vi "AMI_CREA_SECUENCIA_REPITE_NSCAN.vi"(8 "error in (no error)":errorcluster) -> (0 "error out":errorcluster, 3 "SECUENCIA":string[](array[string]), 4 "TOTAL_REPS":string[](array[string]), 6 "PASOS_REPS":i32)   [LabVIEW 2017]
uses:
  <vilib>/Utility/file.llb/Read Delimited Spreadsheet (string).vi
panel:
  out "Array 2":string[](array[string])
  out "PASOS":i32
  out "TOTAL":string[](array[string])
  out "Array":string[][][](array[string])
  out "PASOS_SECUENCIA":i32
  out "End_idx":i32[](array[numeric])
  out "Start_idx":i32[](array[numeric])
  out "Scan X":bool
  out "Scan Y":bool
  out "Scan V":bool
  out "Array2D":string[][](array[string])
  out "Scan T":bool
  out "Scan Z":bool
  in  "Salir":bool
  in  "Borrar línea":bool
  in  "Grabar":bool
  in  "Cargar":bool
  out "SequenceFile":path
  in  "Añadir: (doble click)":i32(listbox) caption="Válvulas"
  in  "Secuencia":i32(listbox)=-1
  # "Ene 2023 V1.6  a_sslcdms"
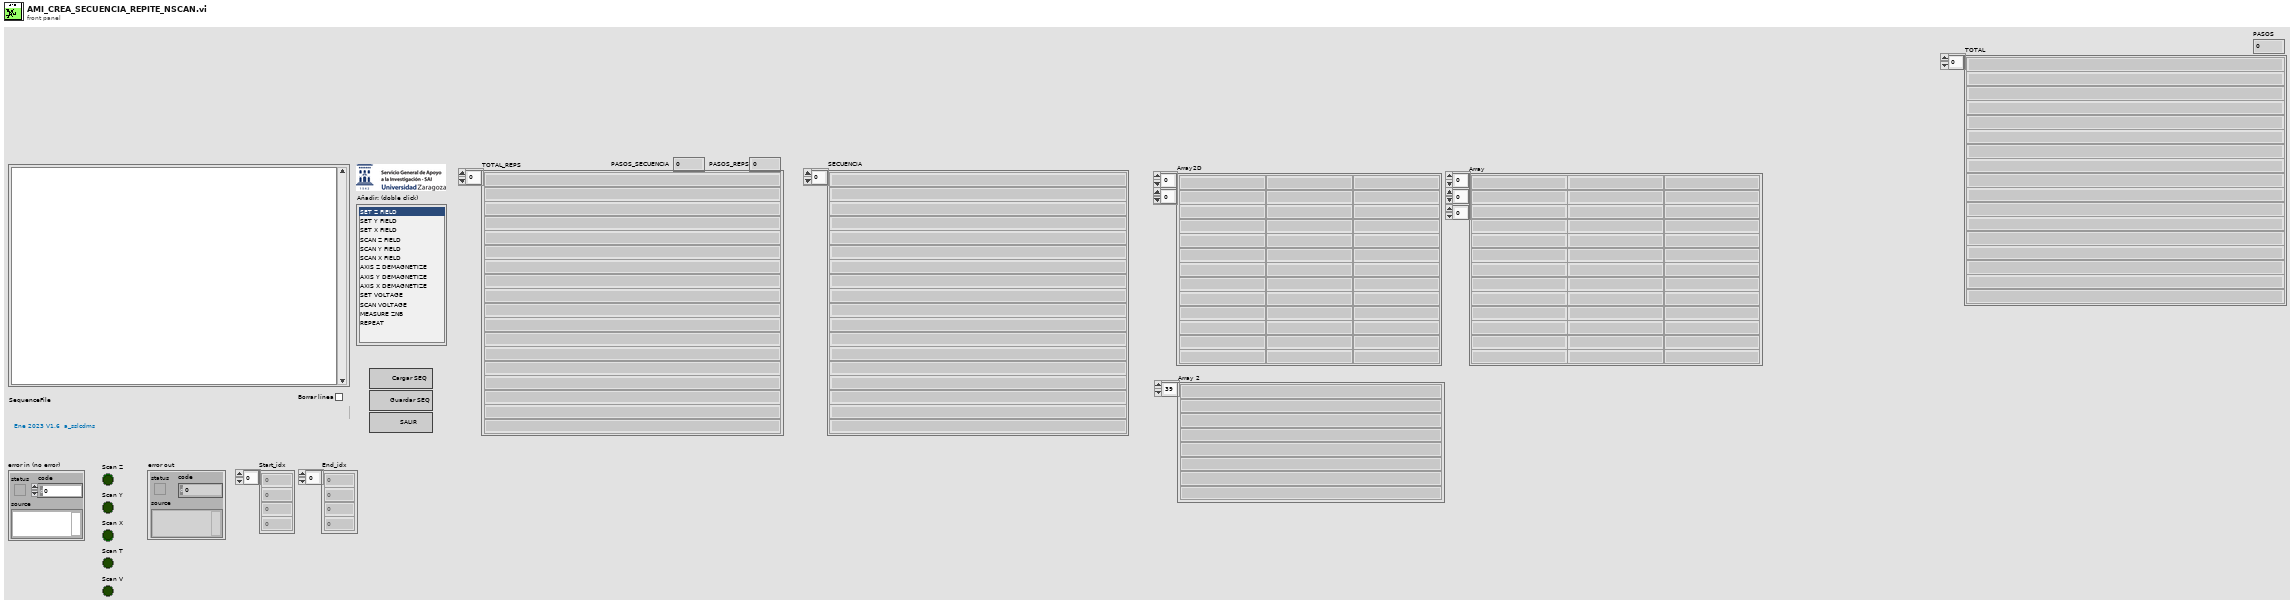
[diagram p1: front panel]
types:
  T1 = enum16{"open", "open or create", "create or replace", "create", "open (read only)"}
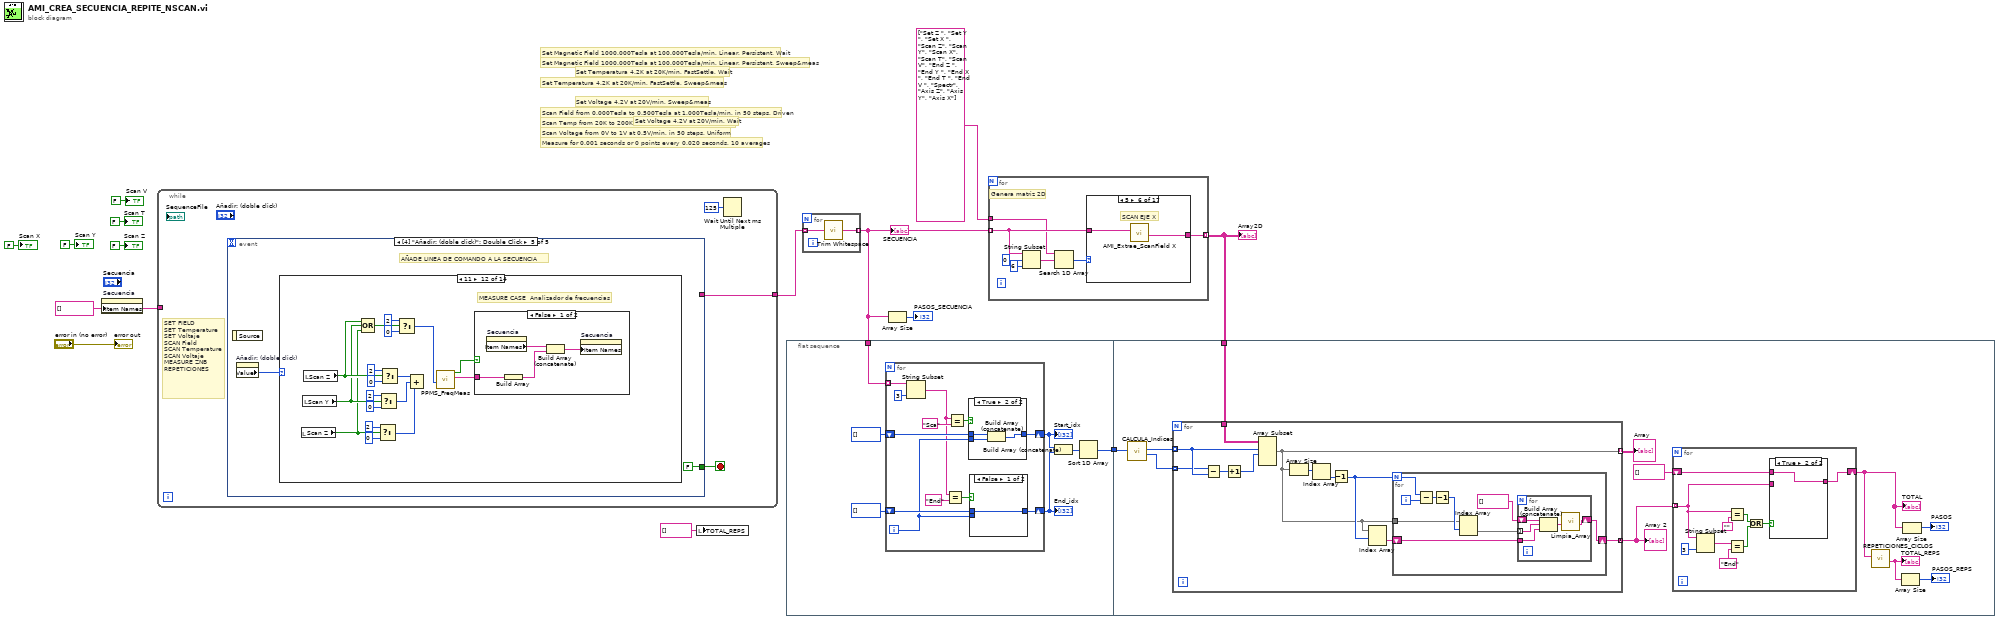
[diagram p0: block diagram]
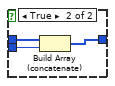
[diagram p2: hidden frame]
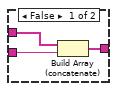
[diagram p4: hidden frame]
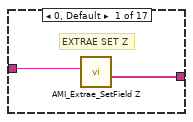
[diagram p5: hidden frame]
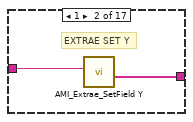
[diagram p6: hidden frame]
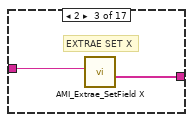
[diagram p7: hidden frame]
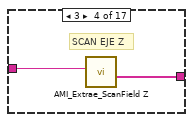
[diagram p8: hidden frame]
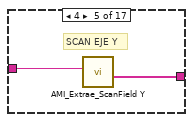
[diagram p9: hidden frame]
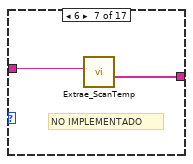
[diagram p10: hidden frame]
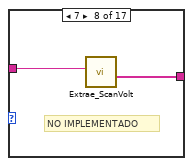
[diagram p11: hidden frame]
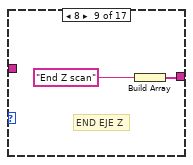
[diagram p12: hidden frame]
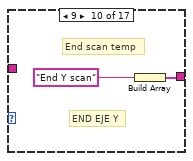
[diagram p13: hidden frame]
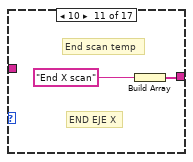
[diagram p14: hidden frame]
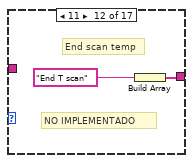
[diagram p15: hidden frame]
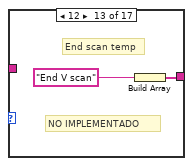
[diagram p16: hidden frame]
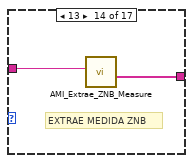
[diagram p17: hidden frame]
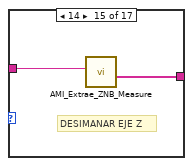
[diagram p18: hidden frame]
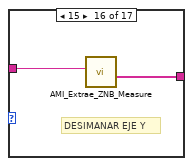
[diagram p19: hidden frame]
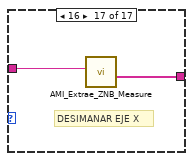
[diagram p20: hidden frame]
diagram:
  w14 = string[] [] ("Item Names")
  # "Measure for 0.001 seconds or 0 points every 0.020 seconds, 10 averages"
  # "Scan Voltage from 0V to 1V at 0.5V/min, in 50 steps, Uniform"
  # "Scan Temp from 20K to 200K at 0.1K/min, in 50 steps, Uniform"
  # "Scan Field from 0.000Tesla to 0.500Tesla at 1.000Tesla/min, in 50 steps, Driven"
  # "Set Temperatura 4.2K at 20K/min, FastSettle, Sweep&meas"
  # "Set Temperatura 4.2K at 20K/min, FastSettle, Wait"
  # "Set Magnetic Field 1000.000Tesla at 100.000Tesla/min, Linear, Persistent, Sweep&meas"
  # "Set Magnetic Field 1000.000Tesla at 100.000Tesla/min, Linear, Persistent, Wait"
  # "Set Voltage 4.2V at 20V/min, Sweep&meas"
  # "Set Voltage 4.2V at 20V/min, Wait"
  n1 = property on="Secuencia" class="LstBox (strict)"("Item Names"=w14) -> ()  [unwired: 2 in, 2 out]
  n2 = while {
    tunnel: w14 -> [_]
    tunnel: [w15] -> w9
    stop <- w16 stop-if-true
    # "SET FIELD\nSET Temperature\nSET Voltaje\nSCAN Field\nSCAN Temperature\nSCAN Voltaje\nMEASURE ZNB\nREPETICIONES"
    n3 = event shown="[4] \"Añadir: (doble click)\": Double Click" {
      selector: _ -> [_ _ _ _ _]
      dyn-events: _ -> [_ _ _ _ _]
      timeout: _ -> [_ _ _ _ _]
      tunnel: [FALSE ("Salir") "Salir" FALSE ("Salir") FALSE ("Salir") FALSE ("Salir")] -> w16
      tunnel: [_ w23 _ _ _] -> w15
      event "Borrar línea": Value Change {
        # "BORRA LA LINEA ACTIVA DE LA SECUENCIA"
        n4 = event-data() -> ()  [unwired: 1 in, 1 out]
        n5 = property on="Secuencia" class="LstBox (strict)"() -> ("Item Names"=w22:string[], "Value"=w21:i32)  [unwired: 2 in, 2 out]
        n6 = Delete From Array(array=w22, length=1, index=w21) -> (array with subset deleted=w19:string[])  [unwired: 1 out]
        n7 = property on="Secuencia" class="LstBox (strict)"("Item Names"=w19) -> ()  [unwired: 2 in, 2 out]
      }
      event "Salir": Value Change {
        # "SALIMOS DEL VI"
        n8 = event-data() -> ()  [unwired: 1 in, 1 out]
        n9 = property on="Secuencia" class="LstBox (strict)"() -> ("Item Names"=w23:string[])  [unwired: 2 in, 2 out]
      }
      event "Cargar": Value Change {
        # "CARGA UNA SECUENCIA ALMACENADA PREVIAMENTE"
        n10 = event-data() -> ()  [unwired: 1 in, 1 out]
        n11 = call-poly <vilib>:"Read Delimited Spreadsheet.vi"() -> ("new file path (Not A Path if cancelled)"=w26:path, "all rows"=w25:string[][])  [unwired: 10 in, 4 out]
        n12 = local write "SequenceFile"(w26) -> ()
        n13 = Index Array(array=w25, index (col)=0 ("disabled index (col)")) -> (element=w27:string[])  [unwired: 1 in]
        n14 = property on="Secuencia" class="LstBox (strict)"("Item Names"=w27) -> ()  [unwired: 2 in, 2 out]
      }
      event "Grabar": Value Change {
        # "GRABA UNA SECUENCIA PARA USAR MAS ADELANTE"
        n15 = event-data() -> ()  [unwired: 1 in, 1 out]
        n16 = property on="Secuencia" class="LstBox (strict)"() -> ("Item Names"=w33:string[])  [unwired: 2 in, 2 out]
        n17 = call <vilib>:"Open_Create_Replace File.vi"("function (open:0)"=T1."create or replace") -> ("new file path"=w30:path)  [unwired: 7 in, 3 out]
        n18 = local write "SequenceFile"(w30) -> ()
        n19 = for {
          tunnel: w33 -> [w36] mode=indexing
          shift-right: [w38] -> _
          shift-left: w30 -> [w39]
          n20 = Concatenate Strings(w36, "\r\n") -> (w35:string)
          n21 = call <vilib>:"Write Characters To File.vi"("append to file? (new file:F)"=TRUE, "character string"=w35, "file path (dialog if empty)"=w39) -> ("new file path (Not A Path if cancelled)"=w38:path)  [unwired: 2 in]
        }
      }
      event "Añadir: (doble click)": Double Click {
        # "AÑADE LINEA DE COMANDO A LA SECUENCIA"
        n22 = event-data() -> ()  [unwired: 1 in, 1 out]
        n23 = property on="Añadir: (doble click)" class="LstBox (strict)"() -> ("Value"=w40:i32)  [unwired: 2 in, 2 out]
        n24 = case shown="11" w40 {
          frame 0, Default {
            # "SET Z FIELD"
            n25 = property on="Secuencia" class="LstBox (strict)"() -> ("Item Names"=w42:string[])  [unwired: 2 in, 2 out]
            n26 = call "AMI_SetCampo Z axis.vi"("Index"=i8 0) -> ("resulting string Z"=w44:string)  [unwired: 7 in, 1 out]
            n27 = Build Array (concatenate)(w42, w44) -> (w43:string[])
            n28 = property on="Secuencia" class="LstBox (strict)"("Item Names"=w43) -> ()  [unwired: 2 in, 2 out]
          }
          frame 1 {
            # "SET Y FIELD"
            n29 = property on="Secuencia" class="LstBox (strict)"() -> ("Item Names"=w47:string[])  [unwired: 2 in, 2 out]
            n30 = call "AMI_SetCampo Y axis.vi"("Index"=i8 0) -> ("resulting string Y"=w49:string)  [unwired: 7 in, 1 out]
            n31 = Build Array (concatenate)(w47, w49) -> (w48:string[])
            n32 = property on="Secuencia" class="LstBox (strict)"("Item Names"=w48) -> ()  [unwired: 2 in, 2 out]
          }
          frame 2 {
            # "SET X FIELD"
            n33 = property on="Secuencia" class="LstBox (strict)"() -> ("Item Names"=w53:string[])  [unwired: 2 in, 2 out]
            n34 = call "AMI_SetCampo X axis.vi"("Index"=i8 0) -> ("resulting string X"=w51:string)  [unwired: 7 in, 1 out]
            n35 = Build Array (concatenate)(w53, w51) -> (w52:string[])
            n36 = property on="Secuencia" class="LstBox (strict)"("Item Names"=w52) -> ()  [unwired: 2 in, 2 out]
          }
          frame 3 {
            # "SCAN Z FIELD"
            n37 = local read "Scan Z"() -> (w55:bool)
            n38 = case shown="False" FALSE {
              tunnel: w55 -> [_ _]
              frame False {
                n39 = local read "Scan X"() -> (w67:bool)
                n40 = local read "Scan Y"() -> (w66:bool)
                n41 = local write "Scan Z"(TRUE ("Scan T")) -> ()
                n42 = Select(t=i8 2 ("Index"), s=w66, f=i8 0 ("Index")) -> (s? t:f=w62:i8)
                n43 = Select(t=i8 2 ("Index"), s=w67, f=i8 0 ("Index")) -> (s? t:f=w63:i8)
                n44 = Add(x=w63, y=w62) -> ()  [unwired: 1 out]
                n45 = call "AMI_ScanCampo Z axis.vi"("Index"=i8 0) -> ("resulting string 2"=w57:string, "resulting string 1"=w56:string)  [unwired: 6 in, 1 out]
                n46 = property on="Secuencia" class="LstBox (strict)"() -> ("Item Names"=w60:string[])  [unwired: 2 in, 2 out]
                n47 = Build Array(w56, w57) -> (w59:string[])
                n48 = Build Array (concatenate)(w60, w59) -> (w58:string[])
                n49 = property on="Secuencia" class="LstBox (strict)"("Item Names"=w58) -> ()  [unwired: 2 in, 2 out]
              }
              frame True {
                n50 = One Button Dialog(message="Solo esta permitido\nun scan de campo por secuencia") -> ()  [unwired: 1 in, 1 out]
              }
            }
          }
          frame 4 {
            # "SCAN Y FIELD"
            n51 = local read "Scan Y"() -> (w73:bool)
            n52 = case shown="False" FALSE {
              tunnel: w73 -> [_ _]
              frame False {
                n53 = local read "Scan X"() -> (w85:bool)
                n54 = local read "Scan Z"() -> (w84:bool)
                n55 = local write "Scan Y"(TRUE ("Scan T")) -> ()
                n56 = Select(t=i8 2 ("Index"), s=w84, f=i8 0 ("Index")) -> (s? t:f=w80:i8)
                n57 = Select(t=i8 2 ("Index"), s=w85, f=i8 0 ("Index")) -> (s? t:f=w81:i8)
                n58 = Add(x=w81, y=w80) -> ()  [unwired: 1 out]
                n59 = call "AMI_ScanCampo Y axis.vi"("Index"=i8 0) -> ("resulting string 2"=w75:string, "resulting string 1"=w74:string)  [unwired: 6 in, 1 out]
                n60 = property on="Secuencia" class="LstBox (strict)"() -> ("Item Names"=w78:string[])  [unwired: 2 in, 2 out]
                n61 = Build Array(w74, w75) -> (w77:string[])
                n62 = Build Array (concatenate)(w78, w77) -> (w76:string[])
                n63 = property on="Secuencia" class="LstBox (strict)"("Item Names"=w76) -> ()  [unwired: 2 in, 2 out]
              }
              frame True {
                n64 = One Button Dialog(message="Solo esta permitido\nun scan de campo por secuencia") -> ()  [unwired: 1 in, 1 out]
              }
            }
          }
          frame 5 {
            # "SCAN X FIELD"
            n65 = local read "Scan X"() -> (w91:bool)
            n66 = case shown="False" FALSE {
              tunnel: w91 -> [_ _]
              frame False {
                n67 = local read "Scan Y"() -> (w103:bool)
                n68 = local read "Scan Z"() -> (w102:bool)
                n69 = local write "Scan X"(TRUE ("Scan T")) -> ()
                n70 = Select(t=i8 2 ("Index"), s=w102, f=i8 0 ("Index")) -> (s? t:f=w98:i8)
                n71 = Select(t=i8 2 ("Index"), s=w103, f=i8 0 ("Index")) -> (s? t:f=w99:i8)
                n72 = Add(x=w99, y=w98) -> ()  [unwired: 1 out]
                n73 = call "AMI_ScanCampo X axis.vi"("Index"=i8 0) -> ("resulting string 2"=w93:string, "resulting string 1"=w92:string)  [unwired: 6 in, 1 out]
                n74 = property on="Secuencia" class="LstBox (strict)"() -> ("Item Names"=w96:string[])  [unwired: 2 in, 2 out]
                n75 = Build Array(w92, w93) -> (w95:string[])
                n76 = Build Array (concatenate)(w96, w95) -> (w94:string[])
                n77 = property on="Secuencia" class="LstBox (strict)"("Item Names"=w94) -> ()  [unwired: 2 in, 2 out]
              }
              frame True {
                n78 = One Button Dialog(message="Solo esta permitido\nun scan de campo por secuencia") -> ()  [unwired: 1 in, 1 out]
              }
            }
          }
          frame 6 {
            # "DESIMANAR Z FIELD"
            n79 = property on="Secuencia" class="LstBox (strict)"() -> ("Item Names"=w108:string[])  [unwired: 2 in, 2 out]
            n80 = call "AMI_Desimana Z axis.vi"("Index"=i8 0) -> ("resulting string Z"=w110:string)  [unwired: 7 in, 1 out]
            n81 = Build Array (concatenate)(w108, w110) -> (w109:string[])
            n82 = property on="Secuencia" class="LstBox (strict)"("Item Names"=w109) -> ()  [unwired: 2 in, 2 out]
          }
          frame 7 {
            # "DESIMANAR Y FIELD"
            n83 = property on="Secuencia" class="LstBox (strict)"() -> ("Item Names"=w113:string[])  [unwired: 2 in, 2 out]
            n84 = call "AMI_Desimana Y axis.vi"("Index"=i8 0) -> ("resulting string Y"=w115:string)  [unwired: 7 in, 1 out]
            n85 = Build Array (concatenate)(w113, w115) -> (w114:string[])
            n86 = property on="Secuencia" class="LstBox (strict)"("Item Names"=w114) -> ()  [unwired: 2 in, 2 out]
          }
          frame 8 {
            # "DESIMANAR X FIELD"
            n87 = property on="Secuencia" class="LstBox (strict)"() -> ("Item Names"=w119:string[])  [unwired: 2 in, 2 out]
            n88 = call "AMI_Desimana X axis.vi"("Index"=i8 0) -> ("resulting string X"=w117:string)  [unwired: 7 in, 1 out]
            n89 = Build Array (concatenate)(w119, w117) -> (w118:string[])
            n90 = property on="Secuencia" class="LstBox (strict)"("Item Names"=w118) -> ()  [unwired: 2 in, 2 out]
          }
          frame 9 {
            # "SET VOLTAGE"
            n91 = case shown="False" FALSE {
              frame False {
                n92 = One Button Dialog(message="Comando desactivado") -> ()  [unwired: 1 in, 1 out]
              }
              frame True {
                n93 = call "PPMS_SetVoltage.vi"("Index"=i8 0) -> ("resulting string 1"=w123:string, "Cancelled?"=w124:bool)  [unwired: 6 in, 1 out]
                n94 = case shown="False" w124 {
                  tunnel: w123 -> [w127 _]
                  frame False {
                    n95 = property on="Secuencia" class="LstBox (strict)"() -> ("Item Names"=w126:string[])  [unwired: 2 in, 2 out]
                    n96 = Build Array (concatenate)(w126, w127) -> (w125:string[])
                    n97 = property on="Secuencia" class="LstBox (strict)"("Item Names"=w125) -> ()  [unwired: 2 in, 2 out]
                  }
                  frame True {
                  }
                }
              }
            }
          }
          frame 10 {
            # "SCAN VOLTAGE"
            n98 = case shown="False" FALSE {
              frame False {
                n99 = One Button Dialog(message="Comando desactivado") -> ()  [unwired: 1 in, 1 out]
              }
              frame True {
                n100 = local read "Scan V"() -> (w130:bool)
                n101 = case shown="False" w130 {
                  frame False {
                    n102 = local read "Scan T"() -> (w138:bool)
                    n103 = local read "Scan Z"() -> (w139:bool)
                    n104 = local write "Scan V"(TRUE ("Scan T")) -> ()
                    n105 = Select(t=i8 2 ("Index"), s=w138, f=i8 0 ("Index")) -> (s? t:f=w136:i8)
                    n106 = Select(t=i8 2 ("Index"), s=w139, f=i8 0 ("Index")) -> (s? t:f=w137:i8)
                    n107 = Add(x=w137, y=w136) -> ()  [unwired: 1 out]
                    n108 = call "PPMS_ScanVoltage.vi"("Index"=i8 0) -> ("resulting string 2"=w141:string, "resulting string 1"=w142:string, "Cancelled?"=w143:bool)  [unwired: 5 in, 1 out]
                    n109 = case shown="False" w143 {
                      tunnel: w142 -> [w148 _]
                      tunnel: w141 -> [w147 _]
                      frame False {
                        n110 = property on="Secuencia" class="LstBox (strict)"() -> ("Item Names"=w146:string[])  [unwired: 2 in, 2 out]
                        n111 = Build Array(w148, w147) -> (w145:string[])
                        n112 = Build Array (concatenate)(w146, w145) -> (w144:string[])
                        n113 = property on="Secuencia" class="LstBox (strict)"("Item Names"=w144) -> ()  [unwired: 2 in, 2 out]
                      }
                      frame True {
                      }
                    }
                  }
                  frame True {
                    n114 = One Button Dialog(message="Solo esta permitido\nun scan de temperatura por secuencia") -> ()  [unwired: 1 in, 1 out]
                  }
                }
              }
            }
          }
          frame 11 {
            # "MEASURE CASE  Analizador de frecuencias"
            n115 = local read "Scan Z"() -> (w154:bool)
            n116 = local read "Scan Y"() -> (w155:bool)
            n117 = local read "Scan Z"() -> (w156:bool)
            n118 = Compound Arithmetic op=OR(w156, w155, w154) -> (w151:bool)
            n119 = Select(t=i8 2 ("Index"), s=w154, f=i8 0 ("Index")) -> (s? t:f=w159:i8)
            n120 = Select(t=i8 2 ("Index"), s=w155, f=i8 0 ("Index")) -> (s? t:f=w162:i8)
            n121 = Select(t=i8 2 ("Index"), s=w156, f=i8 0 ("Index")) -> (s? t:f=w163:i8)
            n122 = Select(t=i8 2 ("Index"), s=w151, f=i8 0 ("Index")) -> (s? t:f=w150:i8)
            n123 = Compound Arithmetic op=ADD(w163, w162, w159) -> ()  [unwired: 1 out]
            n124 = call "PPMS_FreqMeas.vi"("Index"=w150) -> ("resulting string 1"=w157:string, "Cancelled?"=w158:bool)  [unwired: 5 in, 2 out]
            n125 = case shown="False" w158 {
              tunnel: w157 -> [w171 _]
              frame False {
                n126 = property on="Secuencia" class="LstBox (strict)"() -> ("Item Names"=w169:string[])  [unwired: 2 in, 2 out]
                n127 = Build Array(w171) -> (w168:string[])
                n128 = Build Array (concatenate)(w169, w168) -> (w170:string[])
                n129 = property on="Secuencia" class="LstBox (strict)"("Item Names"=w170) -> ()  [unwired: 2 in, 2 out]
              }
              frame True {
              }
            }
          }
          frame 12 {
            n130 = call "PPMS_Repeticiones.vi"() -> ("Ciclos"=w173:i32, "Cancelled?"=w172:bool)  [unwired: 10 in]
            n131 = Format Into String(format string="%s %d %s", "Repetir: " ("input 1"), w173, " veces" ("input 3")) -> (resulting string=w178:string)  [unwired: 2 in, 1 out]
            n132 = case shown="False" w172 {
              tunnel: w178 -> [w182 _]
              tunnel: "Fin repeticiones" ("input 1") -> [w181 _]
              frame False {
                n133 = property on="Secuencia" class="LstBox (strict)"() -> ("Item Names"=w180:string[])  [unwired: 2 in, 2 out]
                n134 = Build Array (concatenate)(w180, w182, w181) -> (w179:string[])
                n135 = property on="Secuencia" class="LstBox (strict)"("Item Names"=w179) -> ()  [unwired: 2 in, 2 out]
              }
              frame True {
              }
            }
          }
          frame 13 {
            # "End Program"
            n136 = property on="Secuencia" class="LstBox (strict)"() -> ("Item Names"=w183:string[])  [unwired: 2 in, 2 out]
            n137 = Build Array (concatenate)(w183, "End Program" ("message")) -> ()  [unwired: 1 out]
            n138 = property on="Secuencia" class="LstBox (strict)"("Item Names"=w183) -> ()  [unwired: 2 in, 2 out]
          }
        }
      }
    }
    n139 = Wait Until Next ms Multiple(millisecond multiple=u32 125) -> ()  [unwired: 1 out]
  }
  n140 = local write "TOTAL_REPS"(string[] [] ("TOTAL_REPS")) -> ()
  n141 = flat-sequence {
    tunnel: w4 -> [w189]
    tunnel: [w185] -> w2
    tunnel: w8 -> [w213]
    tunnel: w2 -> [w220]
    frame #0 {
      n142 = for {
        tunnel: w189 -> [w194] mode=indexing
        shift-right: [w199] -> w187
        shift-left: i32[] [] ("Start") -> [w200]
        shift-right: [w195] -> w186
        shift-left: i32[] [] ("Start") -> [w197]
        i -> [w196]
        n143 = String Subset(string=w194, length (rest)=3 ("length (rest)")) -> (substring=w192:string)  [unwired: 1 in]
        n144 = Equal?(x=w192, y="End" ("trimmed string")) -> (x = y?=w198:bool)
        n145 = Equal?(x=w192, y="Sca" ("trimmed string")) -> (x = y?=w201:bool)
        n146 = case shown="True" w201 {
          tunnel: w200 -> [w208 w210]
          tunnel: [w208 w209] -> w199
          tunnel: w196 -> [_ w211]
          frame False {
          }
          frame True {
            n147 = Build Array (concatenate)(w210, w211) -> (w209:i32[])
          }
        }
        n148 = case shown="False" w198 {
          tunnel: w197 -> [w204 w206]
          tunnel: [w204 w205] -> w195
          tunnel: w196 -> [_ w207]
          frame False {
          }
          frame True {
            n149 = Build Array (concatenate)(w206, w207) -> (w205:i32[])
          }
        }
      }
      "Start_idx" <- w187
      "End_idx" <- w186
      n150 = Build Array (concatenate)(w187, w186) -> (w188:i32[])
      n151 = Sort 1D Array(array=w188) -> (sorted array=w185:i32[])
    }
    frame #1 {
      n152 = call "CALCULA_Indices.vi"("Start_end"=w220) -> ("End 3"=w217:i32[], "Start 3"=w219:i32[])  [unwired: 9 in]
      n153 = for {
        tunnel: w219 -> [w246] mode=indexing
        tunnel: w217 -> [w245] mode=indexing
        tunnel: [w239] -> w218 mode=indexing
        tunnel: [w238] -> w215 mode=concatenating
        tunnel: w213 -> [w237]
        n154 = Subtract(x=w245, y=w246) -> (x-y=w247:i32)
        n155 = Increment(x=w247) -> (x+1=w244:i32)
        n156 = Array Subset(array=w237, index (row)=w246, length (row)=w244) -> (w239:string[][])  [unwired: 2 in]
        n157 = Array Size(array=w239) -> (size(s)=w241:i32[])
        n158 = Index Array(array=w241) -> (element=w242:i32)  [unwired: 1 in]
        n159 = Decrement(x=w242) -> (x-1=w243:i32)
        n160 = Index Array(array=w239, index (row)=w243) -> (element=w240:string[])  [unwired: 1 in]
        n161 = for {
          N: w243 -> [w256]
          tunnel: w239 -> [w253]
          shift-right: [w249] -> w238
          shift-left: w240 -> [w250]
          i -> [w255]
          n162 = Subtract(x=w256, y=w255) -> (x-y=w252:i32)
          n163 = Decrement(x=w252) -> (x-1=w254:i32)
          n164 = Index Array(array=w253, index (row)=w254) -> (element=w248:string[])  [unwired: 1 in]
          n165 = for {
            tunnel: w248 -> [w260] mode=indexing
            shift-right: [w257] -> w249
            shift-left: string[] [] -> [w261]
            tunnel: w250 -> [w259]
            n166 = Build Array (concatenate)(w261, w260, w259) -> (w258:string[])
            n167 = call "Limpia_Array.vi"("Array in"=w258) -> ("Array out"=w257:string[])  [unwired: 10 in]
          }
        }
      }
      "Array" <- w218
      "Array 2" <- w215
      n168 = for {
        tunnel: w215 -> [w224] mode=indexing
        shift-right: [w229] -> w212
        shift-left: string[] [] -> [w230]
        n169 = String Subset(string=w224, length (rest)=3 ("length (rest)")) -> (substring=w227:string)  [unwired: 1 in]
        n170 = Equal?(x=w224, y="") -> (x = y?=w223:bool)
        n171 = Equal?(x=w227, y="End" ("trimmed string")) -> (x = y?=w225:bool)
        n172 = Or(x=w223, y=w225) -> (x .or. y?=w228:bool)
        n173 = case shown="True" w228 {
          tunnel: w230 -> [w235 w236]
          tunnel: [w234 w236] -> w229
          tunnel: w224 -> [w233 _]
          frame False {
            n174 = Build Array (concatenate)(w235, w233) -> (w234:string[])
          }
          frame True {
          }
        }
      }
      "TOTAL" <- w212
      n175 = call "REPETICIONES_CICLOS.vi"("Secuencia"=w212) -> ("Secuciclos"=w222:string[])  [unwired: 9 in, 1 out]
      "TOTAL_REPS" <- w222
      n176 = Array Size(array=w222) -> (size(s)=→"PASOS_REPS":i32)
      n177 = Array Size(array=w212) -> (size(s)=→"PASOS":i32)
    }
  }
  n178 = for {
    tunnel: w9 -> [w263] mode=indexing
    tunnel: [w262] -> w4 mode=indexing
    n179 = call <vilib>:"Trim Whitespace.vi"("string"=w263) -> ("trimmed string"=w262:string)  [unwired: 1 in]
  }
  "SECUENCIA" <- w4
  n180 = Array Size(array=w4) -> (size(s)=→"PASOS_SECUENCIA":i32)
  n181 = for {
    tunnel: w4 -> [w266] mode=indexing
    tunnel: [w264] -> w8 mode=indexing
    tunnel: string[] ["Set Z ", "Set Y ", "Set X ", "Scan Z", "Scan Y", "Scan X", "Scan T", "Scan V", "End Z ", "End Y ", "End X ", "End T ", "End V ", "Spectr", "Axis Z", "Axis Y", "Axis X"] ("Array") -> [w265]
    # "Genera matriz 2D"
    n182 = String Subset(string=w266, offset (0)=0, length (rest)=6 ("length (rest)")) -> (substring=w268:string)
    n183 = Search 1D Array(1D array=w265, element=w268) -> (index of element=w267:i32)  [unwired: 1 in]
    n184 = case shown="5" w267 {
      tunnel: w266 -> [w272 w274 w276 w278 w280 w282 w284 w286 _ _ _ _ _ w298 w300 w302 w304]
      tunnel: [w271 w273 w275 w277 w279 w281 w283 w285 w287 w289 w291 w293 w295 w297 w299 w301 w303] -> w264
      frame 0, Default {
        # "EXTRAE SET Z"
        n185 = call "AMI_Extrae_SetField Z.vi"("String"=w272) -> ("Array"=w271:string[])  [unwired: 10 in]
      }
      frame 1 {
        # "EXTRAE SET Y"
        n186 = call "AMI_Extrae_SetField Y.vi"("String"=w274) -> ("Array"=w273:string[])  [unwired: 10 in]
      }
      frame 2 {
        # "EXTRAE SET X"
        n187 = call "AMI_Extrae_SetField X.vi"("String"=w276) -> ("Array"=w275:string[])  [unwired: 10 in]
      }
      frame 3 {
        # "SCAN EJE Z"
        n188 = call "AMI_Extrae_ScanField Z.vi"("F string"=w278) -> ("Array F"=w277:string[])  [unwired: 10 in]
      }
      frame 4 {
        # "SCAN EJE Y"
        n189 = call "AMI_Extrae_ScanField Y.vi"("F string"=w280) -> ("Array F"=w279:string[])  [unwired: 10 in]
      }
      frame 5 {
        # "SCAN EJE X"
        n190 = call "AMI_Extrae_ScanField X.vi"("F string"=w282) -> ("Array F"=w281:string[])  [unwired: 10 in]
      }
      frame 6 {
        # "NO IMPLEMENTADO"
        n191 = call "Extrae_ScanTemp.vi"("T string"=w284) -> ("Array T"=w283:string[])  [unwired: 10 in]
      }
      frame 7 {
        # "NO IMPLEMENTADO"
        n192 = call "Extrae_ScanVolt.vi"("V string"=w286) -> ("Array V"=w285:string[])  [unwired: 10 in]
      }
      frame 8 {
        # "END EJE Z"
        n193 = Build Array("End Z scan" ("trimmed string")) -> (w287:string[])
      }
      frame 9 {
        # "END EJE Y"
        # "End scan temp"
        n194 = Build Array("End Y scan" ("trimmed string")) -> (w289:string[])
      }
      frame 10 {
        # "END EJE X"
        # "End scan temp"
        n195 = Build Array("End X scan" ("trimmed string")) -> (w291:string[])
      }
      frame 11 {
        # "NO IMPLEMENTADO"
        # "End scan temp"
        n196 = Build Array("End T scan" ("trimmed string")) -> (w293:string[])
      }
      frame 12 {
        # "NO IMPLEMENTADO"
        # "End scan temp"
        n197 = Build Array("End V scan" ("trimmed string")) -> (w295:string[])
      }
      frame 13 {
        # "EXTRAE MEDIDA ZNB"
        n198 = call "AMI_Extrae_ZNB_Measure.vi"("String"=w298) -> ("Array"=w297:string[])  [unwired: 10 in]
      }
      frame 14 {
        # "DESIMANAR EJE Z"
        n199 = call "AMI_Extrae_ZNB_Measure.vi"("String"=w300) -> ("Array"=w299:string[])  [unwired: 10 in]
      }
      frame 15 {
        # "DESIMANAR EJE Y"
        n200 = call "AMI_Extrae_ZNB_Measure.vi"("String"=w302) -> ("Array"=w301:string[])  [unwired: 10 in]
      }
      frame 16 {
        # "DESIMANAR EJE X"
        n201 = call "AMI_Extrae_ZNB_Measure.vi"("String"=w304) -> ("Array"=w303:string[])  [unwired: 10 in]
      }
    }
  }
  "Array2D" <- w8
  "error out" <- "error in (no error)"
  "Scan Z" <- FALSE ("Loop H")
  "Scan T" <- FALSE ("Loop T")
  "Scan V" <- FALSE ("Loop T")
  "Scan Y" <- FALSE ("Loop H")
  "Scan X" <- FALSE ("Loop H")
